vi "Poll Sensor.vi"(8 "error in":errorcluster, 9 "Sensor ID":T2, 11 "UART port in":T1) -> (0 "error out":errorcluster, 3 "UART port out":T1)   [LabVIEW 2014]
doc: "Request a single sensor packet. Returns immediately after requesting; bytes must be read off of the UART port and processed to receive the packet.\n\nThis VI writes to, but does not read from, the serial port."
uses:
  Sensor ID.ctl
  Advanced/UART/iRobot UART Port Type.ctl
  Advanced/Command/OpCode.ctl
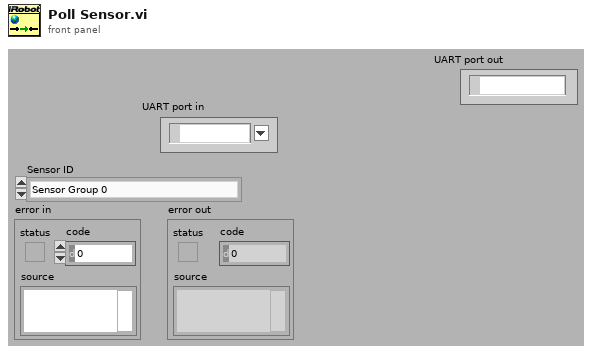
[diagram p1: front panel]
types:
  T1 = typedef "iRobot UART Port Type.ctl" = refnum<visa-resource-name>
  T2 = typedef "Sensor ID.ctl" = enum8{"Sensor Group 0", "Sensor Group 1", "Sensor Group 2", "Sensor Group 3", "Sensor Group 4", "Sensor Group 5", "Sensor Group 6", "Bump + Wheel Drop", "Wall", "Cliff Left", "Cliff Front Left", "Cliff Front Right", "Cliff Right", "Virtual Wall", "Low Side Driver + Wheel Overcurrent", "Unused 0", "Unused 1", "Infrared", "Buttons", "Distance", "Angle", "Charging State", "Voltage", "Current", "Battery Temperature", "Battery Charge", "Battery Capacity", "Wall Signal", "Cliff Left Signal", "Cliff Front Left Signal", "Cliff Front Right Signal", "Cliff Right Signal", "Cargo Bay Digital Inputs", "Cargo Bay Analog Signal", "Charging Sources Available", "OI Mode", "Song Number", "Song Playing", "Number of Stream Packets", "Requested Velocity", "Requested Radius", "Requested Right Velocity", "Requested Left Velocity"}
  T3 = typedef "OpCode.ctl" = u8
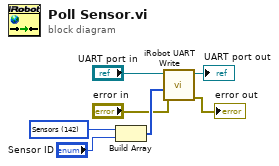
[diagram p0: block diagram]
diagram:
  w7 = T3 142 items=["Start"=128, "Baud"=129, "Control"=130, "Safe"=131, "Full"=132, "Demo"=136, "Demo - Cover"=135, "Demo - Cover and Dock"=143, "Demo - Spot"=134, "Drive"=137, "Drive Direct"=145, "LEDs"=139, "Digital Outputs"=147, "PWM Low Side Drivers"=144, "Low Side Drivers"=138, "Send IR"=151, "Song"=140, "Play Song"=141, "Sensors"=142, "Query List"=149, "Stream"=148, "Pause/Resume Stream"=150, "Script"=152, "Play Script"=153, "Show Script"=154, "Wait Time"=155, "Wait Distance"=156, "Wait Angle"=157, "Wait Event"=158] ("OpCode")
  n1 = Build Array(w7, "Sensor ID") -> (w5:T3[])
  n2 = call "iRobot UART Write.vi"("error in"="error in", "data"=w5, "UART port in"="UART port in") -> ("error out"=→"error out":errorcluster, "UART port out"=→"UART port out":T1)  [unwired: 1 in, 6 out]
